vi "Load Streamed Data.vi"(0 "# Records (-1)":i32=-1, 1 "# Records to Skip":i32, 2 "Source File":path=path "C:/ScopeBinaryData.bin", 3 "# Channels":i32=7, 4 "Samples per Record":i32=51200) -> (5 "Array":dbl[][](array[numeric]))   [LabVIEW 2013]
panel:
  out "Waveform Graph":dbl[][](graph)
  out "# Records to be Read":i64
  out "num elements read":i32
  out "Size":i32[](array[numeric])
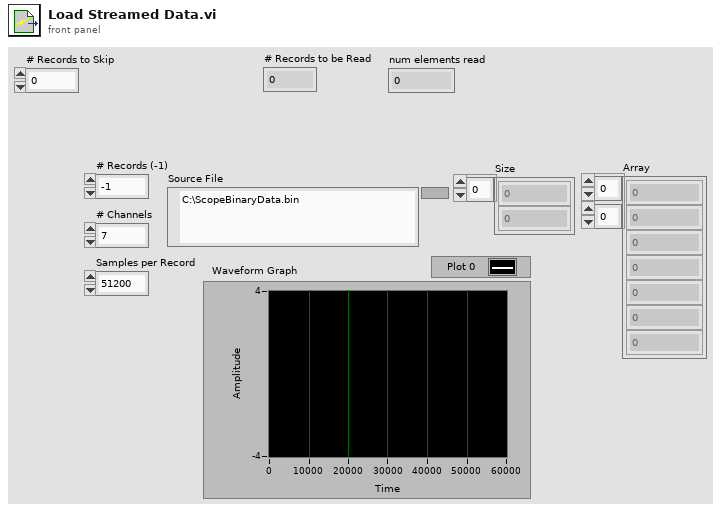
[diagram p1: front panel]
types:
  T1 = enum32{"CREATE_NEW (create)", "CREATE_ALWAYS (replace or create)", "OPEN_EXISTING (open)", "OPEN_ALWAYS (open or create)", "TRUNCATE_EXISTING (replace)"}
  T2 = enum16{"big-endian, network order", "native, host order", "little-endian"}
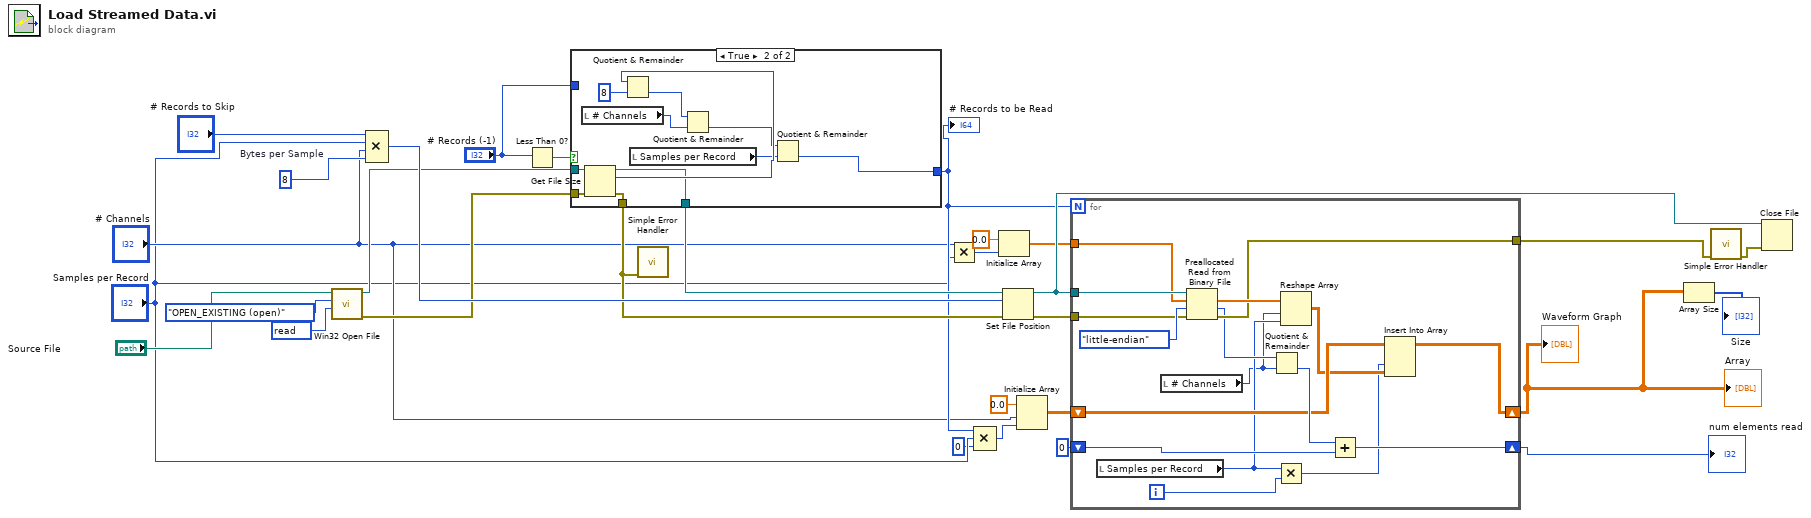
[diagram p0: block diagram]
diagram:
  w23 = 8  # Bytes per Sample
  w29 = u32 2147483648 items=["read"=2147483648, "write"=1073741824, "read & write"=3221225472, "execute"=536870912, "all"=268435456] ("desired access (read & write)")
  n1 = call "Win32 Open File.vi"("desired access (read & write)"=w29, "creation mode (open)"=T1."OPEN_EXISTING (open)", "file path"="Source File") -> ("error out"=w17:errorcluster, "LabVIEW file refnum out"=w18:refnum<file>)  [unwired: 6 in, 1 out]
  n2 = Compound Arithmetic op=MULTIPLY("# Records to Skip", "Samples per Record", "# Channels", w23) -> (w22:i32)
  n3 = Less Than 0?(x="# Records (-1)") -> (x < 0?=w19:bool)
  n4 = case shown="True" w19 {
    tunnel: w18 -> [w32 w44]
    tunnel: w17 -> [w31 w43]
    tunnel: "# Records (-1)" -> [w33 _]
    tunnel: [w33 w38] -> w10
    tunnel: [w32 w37] -> w15
    tunnel: [w31 w36] -> w14
    frame False {
    }
    frame True {
      n5 = local read "# Channels"() -> (w39:i32)
      n6 = Get File Size(file=w44, error in=w43) -> (refnum out=w37:refnum<file>, size (in bytes)=w42:i64, 0:w36:errorcluster)
      n7 = Quotient & Remainder(x=w42, y=i64 8) -> (floor(x/y)=w40:i64)  [unwired: 1 out]
      n8 = local read "Samples per Record"() -> (w34:i32)
      n9 = Quotient & Remainder(x=w40, y=w39) -> (floor(x/y)=w35:i64)  [unwired: 1 out]
      n10 = Quotient & Remainder(x=w35, y=w34) -> (floor(x/y)=w38:i64)  [unwired: 1 out]
    }
  }
  "# Records to be Read" <- w10
  n11 = call <vilib>:"Simple Error Handler.vi"("error in (no error)"=w14) -> ()  [unwired: 4 in, 5 out]
  n12 = Multiply(x="# Channels", y="Samples per Record") -> (x*y=w7:i32)
  n13 = Compound Arithmetic op=MULTIPLY(w10, "Samples per Record", 0 ("value")) -> (w9:i64)
  n14 = Initialize Array(0.0 ("element"), w7) -> (w4:dbl[])
  n15 = Set File Position(offset (in bytes) (0)=w22, refnum=w15, error in=w14) -> (refnum out=w11:refnum<file>, error out=w25:errorcluster)  [unwired: 1 in]
  n16 = Initialize Array(0.0 ("element"), "# Channels", w9) -> (w2:dbl[][])
  n17 = for {
    N: w10 -> [_]
    tunnel: w11 -> [w59]
    tunnel: w25 -> [w60]
    tunnel: w4 -> [w58]
    tunnel: [w56] -> w13
    shift-right: [w54] -> w20
    shift-left: 0 ("num elements read") -> [w52]
    shift-right: [w49] -> w1
    shift-left: w2 -> [w51]
    i -> [w50]
    n18 = local read "Samples per Record"() -> (w46:i32)
    n19 = local read "# Channels"() -> (w45:i32)
    n20 = Preallocated Read from Binary File(4:w60, 5:T2."little-endian" ("byte order (0:big-endian, network order)"), 6:w58, 7:w59) -> (0:w56:errorcluster, 1:w55:i32, 2:w57:dbl[])  [unwired: 1 out]
    n21 = Quotient & Remainder(x=w55, y=w45) -> (floor(x/y)=w53:i32)  [unwired: 1 out]
    n22 = Multiply(x=w46, y=w50) -> (x*y=w47:i32)
    n23 = Reshape Array(w57, w45, w46) -> (w48:dbl[][])
    n24 = Add(x=w53, y=w52) -> (x+y=w54:i32)
    n25 = Insert Into Array(array=w51, index (col)=w47, new element=w48) -> (w49:dbl[][])  [unwired: 1 in]
  }
  "Array" <- w1
  "num elements read" <- w20
  "Waveform Graph" <- w1
  n26 = Array Size(array=w1) -> (size(s)=→"Size":i32[])
  n27 = call <vilib>:"Simple Error Handler.vi"("error in (no error)"=w13) -> ("error out"=w12:errorcluster)  [unwired: 4 in, 4 out]
  n28 = Close File(refnum=w11, error in=w12) -> ()  [unwired: 2 out]
